vi "Sub-Panel Test.vi"() -> ()   [LabVIEW 2017]
uses:
  DSF Mini Explorer.vi
  DSF Mini Explorer.lvlib
panel:
  in  "stop":bool
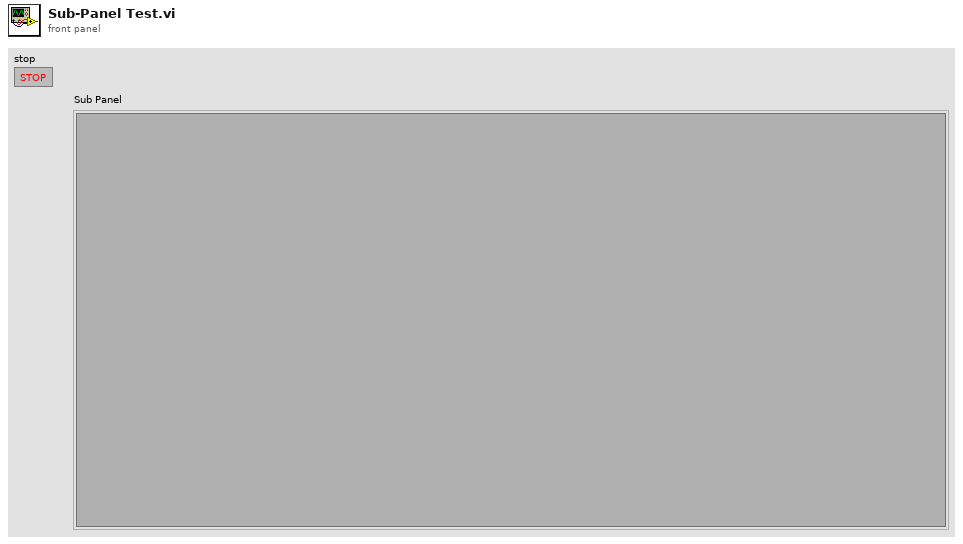
[diagram p1: front panel]
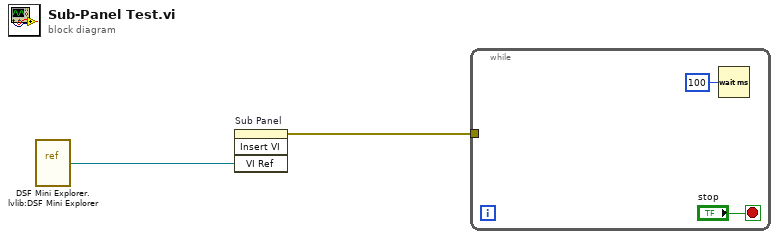
[diagram p0: block diagram]
diagram:
  n1 = vi-ref "DSF Mini Explorer.lvlib:DSF Mini Explorer.vi"() -> (w1:refnum<vi>)
  n2 = invoke on="Sub Panel" class="SubPnl" method="Insert VI"("VI Ref"=w1) -> (error out=w2:errorcluster)  [unwired: 3 in, 3 out]
  n3 = while {
    tunnel: w2 -> [_]
    stop <- "stop" stop-if-true
    n4 = Wait (ms)(milliseconds to wait=u32 100) -> ()  [unwired: 1 out]
  }
